vi "Configure Display.vi"(6 "Display Setup Commands":T1={"Mode (0: Measurement Input)"=0, "Num Fields (0: 2 Large)"=0, "Displayed Info (1: Sample Heater)"=1} {"Displayed Info (1: Sample Heater)" items=["None", "Sample Heater", "Warm-up Heater", "Active Scan Channel"]; "Num Fields (0: 2 Large)" items=["2 Large", "4 Large", "8 Small"]; "Mode (0: Measurement Input)" items=["Measurement Input", "Control Input", "Custom"]}, 7 "Display Field Parameters":T2={"Field (Location)"=1, "Channel (1:1)"=1, "Source (2: Ohms)"=2} {"Source (2: Ohms)" items=["Kelvin"=1, "Ohms"=2, "Quadrature"=3, "Min Data"=4, "Max Data"=5, "Sensor Name"=6]; "Channel (1:1)" items=["All Channels", "1", "2", "3", "4", "5", "6", "7", "8", "9", "10", "11", "12", "13", "14", "15", "16", "A (Control Input)"]; "Field (Location)" min=1 max=8 step=1}, 8 "error in (no error)":errorcluster, 9 "LEDs On (Off)":bool, 10 "Display Brightness (1: 50%)":u16(ring)=1 items=["25%", "50%", "75%", "100%"], 11 "VISA resource name":refnum<visa-resource-name>) -> (0 "error out":errorcluster, 3 "VISA resource name out":refnum<visa-resource-name>)   [LabVIEW 2018, in "Lake Shore 372.lvlib"]
doc: "Configures the parameters of the front panel display. Commands used are <B>BRIGT</B>, <B>DISPLAY</B>, <B>DISPFLD</B>, and <B>LEDS</B>."
uses:
  Lake Shore 372.lvlib
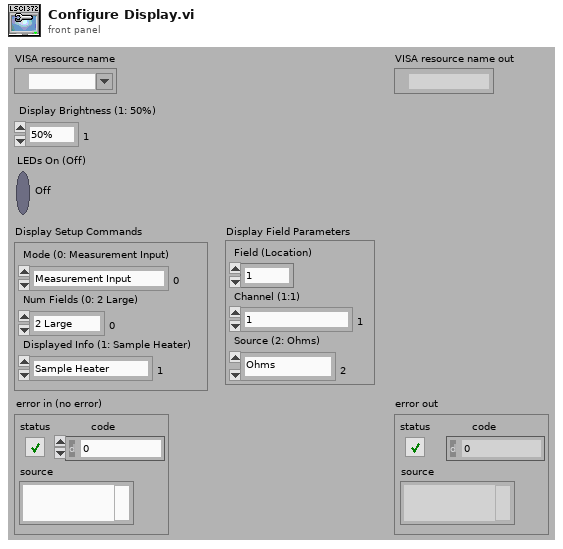
[diagram p1: front panel]
types:
  T1 = cluster{"Mode (0: Measurement Input)":u16, "Num Fields (0: 2 Large)":u16, "Displayed Info (1: Sample Heater)":u16}
  T2 = cluster{"Field (Location)":i32, "Channel (1:1)":u16, "Source (2: Ohms)":u16}
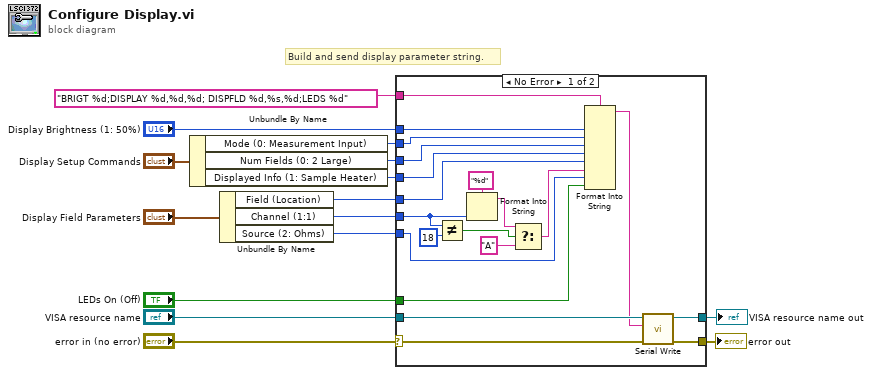
[diagram p0: block diagram]
diagram:
  # "Build and send display parameter string."
  n1 = Unbundle By Name("Display Setup Commands") -> ("Mode (0: Measurement Input)"=w6:u16, "Num Fields (0: 2 Large)"=w5:u16, "Displayed Info (1: Sample Heater)"=w4:u16)
  n2 = Unbundle By Name("Display Field Parameters") -> ("Field (Location)"=w3:i32, "Channel (1:1)"=w2:u16, "Source (2: Ohms)"=w1:u16)
  n3 = case shown="No Error" "error in (no error)" {
    selector: "error in (no error)" -> [w29 w36]
    tunnel: "VISA resource name" -> [w35 w37]
    tunnel: [w34 w37] -> w14
    tunnel: [w33 w36] -> w13
    tunnel: "BRIGT %d;DISPLAY %d,%d,%d; DISPFLD %d,%s,%d;LEDS %d" -> [w32 _]
    tunnel: "Display Brightness (1: 50%)" -> [w31 _]
    tunnel: w6 -> [w28 _]
    tunnel: w5 -> [w27 _]
    tunnel: w4 -> [w26 _]
    tunnel: "LEDs On (Off)" -> [w16 _]
    tunnel: w3 -> [w25 _]
    tunnel: w2 -> [w20 _]
    tunnel: w1 -> [w24 _]
    frame No Error {
      n4 = Not Equal?(x=w20, y=18) -> (x != y?=w22:bool)
      n5 = Format Into String(format string="%d", w20) -> (resulting string=w19:string)  [unwired: 2 in, 1 out]
      n6 = Select(t=w19, s=w22, f="A") -> (s? t:f=w17:string)
      n7 = Format Into String(format string=w32, w31, w28, w27, w26, w25, w17, w24, w16) -> (resulting string=w30:string)  [unwired: 2 in, 1 out]
      n8 = call "Serial Write.vi"("error in (no error)"=w29, "Write Buffer (\"\")"=w30, "VISA resource name"=w35) -> ("error out"=w33:errorcluster, "VISA resource name out"=w34:refnum<visa-resource-name>)  [unwired: 6 in, 1 out]
    }
    frame Error {
    }
  }
  "error out" <- w13
  "VISA resource name out" <- w14
